vi "start_pulse_task.vi"(8 "error in":errorcluster, 11 "Clock In":refnum<class "ClockDL100201DAQmx.lvclass">) -> (0 "error out":errorcluster, 3 "Clock Out":refnum<class "ClockDL100201DAQmx.lvclass">)   [LabVIEW 2010, in "ClockDL100201DAQmx.lvclass"]
doc: "This vi configures and starts the pulse train output task. Output of this task is triggered by the signal of the period task."
uses:
  ClockDL100201DAQmx.lvclass
  ClockDL100201DAQmx.lvclass/ClockDL100201DAQmx.ctl
  <vilib>/DAQmx/write.llb/DAQmx Write (Digital 1D U8 1Chan NSamp).vi
  <vilib>/DAQmx/create/channels.llb/DAQmx Create Channel (DO-Digital Output).vi
  <vilib>/DAQmx/configure/timing.llb/DAQmx Timing (Sample Clock).vi
  <vilib>/DAQmx/configure/trigger.llb/DAQmx Start Trigger (Digital Edge).vi
  <vilib>/daqmx/miscellaneous.llb/DAQmx Fill In Error Info.vi
  Program Files (x86)/National Instruments/LabVIEW 2010/resource/objmgr/daqmx.rc
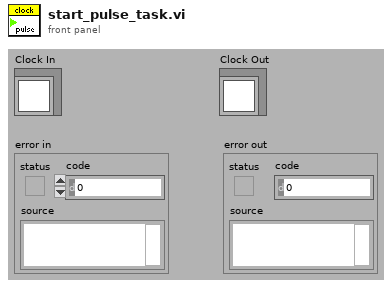
[diagram p1: front panel]
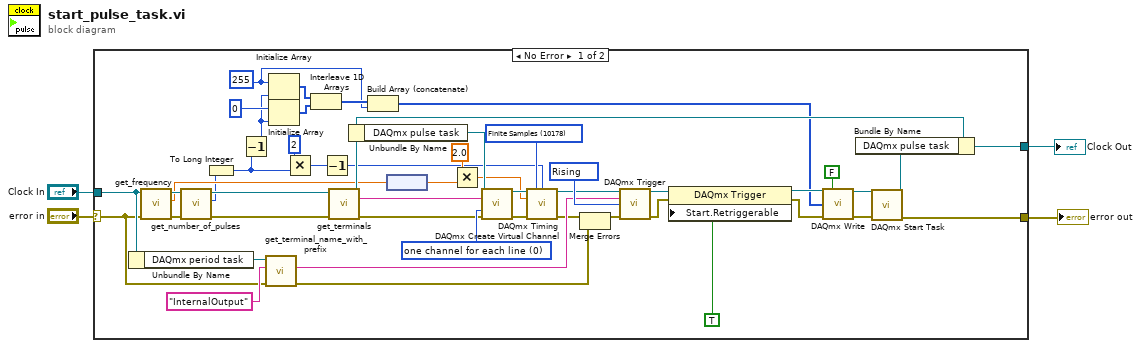
[diagram p0: block diagram]
diagram:
  n1 = case shown="No Error" "error in" {
    selector: "error in" -> [w38 w54]
    tunnel: "Clock In" -> [w48 w55]
    tunnel: [w18 w54] -> w3
    tunnel: [w46 w55] -> w2
    frame No Error {
      w7 = u8 255
      w37 = 0 items=["one channel for each line", "one channel for all lines"] ("line grouping")
      w53 = 10280 items=["Rising"=10280, "Falling"=10171] ("edge")
      w39 = 10178 items=["Finite Samples"=10178, "Continuous Samples"=10123, "Hardware Timed Single Point"=12522] ("sample mode")
      n2 = Unbundle By Name(w48) -> ("DAQmx period task"=w49:refnum<k21>)
      n3 = call-dynamic "get_frequency.vi"("error in (no error)"=w38, "GenericClock.lvclass in"=w48) -> ("error out"=w43:errorcluster, "frequency"=w36:dbl[unit], "GenericClock.lvclass out"=w44:refnum<class "ClockDL100201DAQmx.lvclass">)  [unwired: 7 in]
      n4 = call-dynamic "get_number_of_pulses.vi"("error in (no error)"=w43, "GenericClock.lvclass in"=w44) -> ("error out"=w25:errorcluster, "number of pulses"=w11:i64, "GenericClock.lvclass out"=w26:refnum<class "ClockDL100201DAQmx.lvclass">)  [unwired: 7 in]
      n5 = To Long Integer(number=w11) -> (32bit integer=w9:i32)
      n6 = Decrement(x=w9) -> (x-1=w10:i32)
      n7 = call "get_terminal_name_with_prefix.vi"("error in (no error)"=w38, "Local Terminal Name"="InternalOutput", "task in"=w49) -> ("error out"=w51:errorcluster, "Terminal Name with Device Prefix"=w52:tag)  [unwired: 6 in, 1 out]
      n8 = Initialize Array(w7, w10) -> (w29:u8[])
      n9 = Initialize Array(u8 0, w10) -> (w28:u8[])
      n10 = Multiply(x=2, y=w9) -> (x*y=w31:i32)
      n11 = Interleave 1D Arrays(w29, w28) -> (w8:u8[])
      n12 = Decrement(x=w31) -> (x-1=w5:i32)
      n13 = call-dynamic "get_terminals.vi"("ClockDL100201DAQmx in"=w26, "error in (no error)"=w25) -> ("ClockDL100201DAQmx out"=w45:refnum<class "ClockDL100201DAQmx.lvclass">, "output terminal"=w24:tag, "error out"=w23:errorcluster)  [unwired: 9 in, 2 out]
      n14 = Unbundle By Name(w45) -> ("DAQmx pulse task"=w47:refnum<k21>)
      n15 = Build Array (concatenate)(w8, w7) -> (w6:u8[])
      n16 = node(w36) -> (w34:dbl)
      n17 = Multiply(x=2.0 ("y"), y=w34) -> (x*y=w35:dbl)
      n18 = call-poly <vilib>:"DAQmx Create Virtual Channel.vi"("task in"=w47, "lines"=w24, "line grouping"=w37, "error in"=w23) -> ("task out"=w40:refnum<k21>, "error out"=w41:errorcluster)  [unwired: 10 in]
      n19 = call-poly <vilib>:"DAQmx Timing.vi"("task/channels in"=w40, "sample mode"=w39, "samples per channel"=w5, "rate"=w35, "error in"=w41) -> ("task out"=w42:refnum<k21>, "error out"=w22:errorcluster)  [unwired: 9 in]
      n20 = Merge Errors(w22, w51) -> (w21:errorcluster)
      n21 = call-poly <vilib>:"DAQmx Trigger.vi"("task/channels in"=w42, "source"=w52, "edge"=w53, "error in"=w21) -> ("task out"=w17:refnum<k21>, "error out"=w16:errorcluster)  [unwired: 10 in]
      n22 = property class="DAQmx Trigger"(reference=w17, error in=w16, "Start.Retriggerable"=TRUE) -> (reference out=w14:refnum<k21>, error out=w15:errorcluster)
      n23 = call-poly <vilib>:"DAQmx Write.vi"("task/channels in"=w14, "auto start"=FALSE, "data"=w6, "error in"=w15) -> ("task out"=w13:refnum<k21>, "error out"=w12:errorcluster)  [unwired: 9 in, 1 out]
      n24 = call <vilib>:"DAQmx Start Task.vi"("task/channels in"=w13, "error in"=w12) -> ("task out"=w19:refnum<k21>, "error out"=w18:errorcluster)  [unwired: 12 in]
      n25 = Bundle By Name(cluster=w45, "DAQmx pulse task"=w19) -> (w46:refnum<class "ClockDL100201DAQmx.lvclass">)
    }
    frame Error {
    }
  }
  "error out" <- w3
  "Clock Out" <- w2
